vi "peak and level crossings.vi"() -> ()   [LabVIEW 2017]
uses:
  <vilib>/Analysis/1siggen.llb/Ramp Pattern by Delta.vi
  <vilib>/Analysis/NI_AALBase.lvlib
panel:
  out "XY Graph":cluster{dbl[], "Amplitudes":dbl[]}[](graph)
  out "peak locations":dbl[](array[numeric])
  out "mean of peaks":dbl format="%0.2f"
  out "crossing":dbl[](array[numeric])
  in  "threshold":dbl=0.4 format="%0.2f"
  in  "end":dbl=256.0
  in  "crossing level":dbl
  in  "width":i32=3 min=3
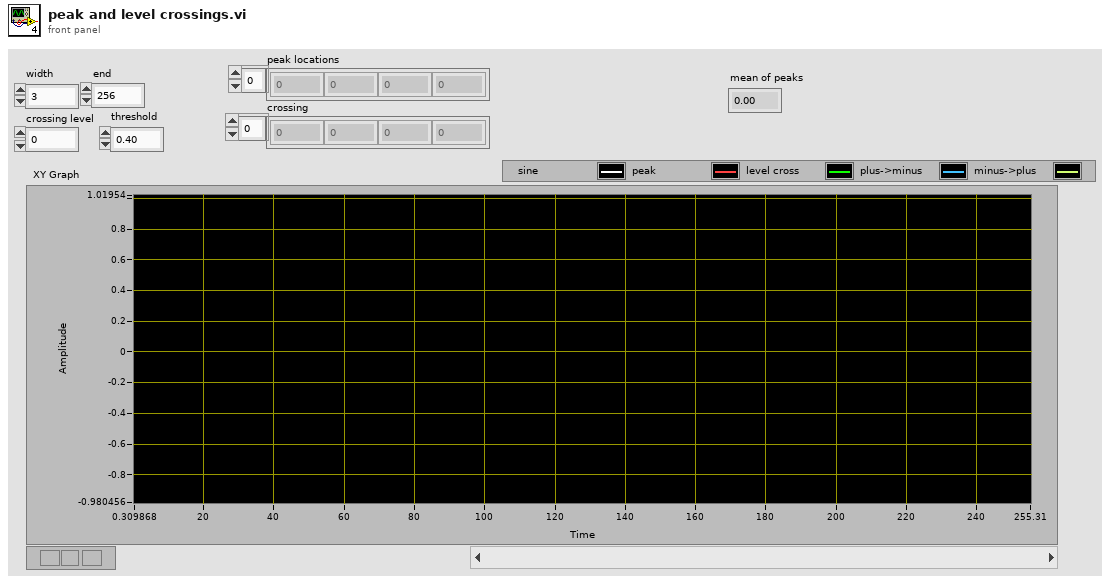
[diagram p1: front panel]
types:
  T1 = cluster{"Ramp Pattern":dbl[], "Amplitudes":dbl[]}[]
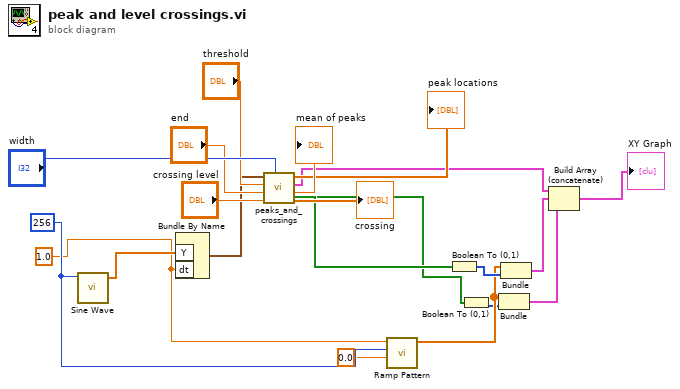
[diagram p0: block diagram]
diagram:
  w2 = 1.0 ("amplitude")
  w12 = 256 ("samples")
  n1 = call <vilib>:"Sine Wave.vi"("samples"=w12) -> ("sine wave"=w13:dbl[])  [unwired: 4 in, 2 out]
  n2 = Bundle By Name("Y"=w13, "dt"=w2) -> (w14:waveform(dbl))  [unwired: 1 in]
  n3 = call "peaks_and_crossings.vi"("width"="width", "crossing level"="crossing level", "end"="end", "threshold"="threshold", "waveform"=w14) -> ("crossing"=→"crossing":dbl[], "mean of peaks"=→"mean of peaks":dbl, "all in array"=w5:cluster{dbl[], "Amplitudes":dbl[]}[], "peak locations"=→"peak locations":dbl[], "plus-minus"=w10:bool[], "minus-plus"=w7:bool[])  [unwired: 1 out]
  n4 = call-poly <vilib>:"Ramp Pattern.vi"("start"=0.0, "end"=w12, "delta"=w2) -> ("Ramp Pattern"=w9:dbl[])  [unwired: 6 in, 2 out]
  n5 = Boolean To (0,1)(Boolean=w10) -> (0, 1=w11:i16[])
  n6 = Boolean To (0,1)(Boolean=w7) -> (0, 1=w8:i16[])
  n7 = Bundle("Ramp Pattern"=w9, w8) -> (w3:cluster{"Ramp Pattern":dbl[], i16[]})  [unwired: 1 in]
  n8 = Bundle("Ramp Pattern"=w9, w11) -> (w4:cluster{"Ramp Pattern":dbl[], i16[]})  [unwired: 1 in]
  n9 = Build Array (concatenate)(w5, w4, w3) -> (→"XY Graph":T1)
